vi "ManualScan-V17.vi"(8 "Button-OK":bool, 10 "menu reference":refnum<k9>, 11 "SN Length":string) -> (1 "MainProcess":T1, 3 "Barcode out:":string)   [LabVIEW 2013]
uses:
  Control/SystemProcess.ctl
  <vilib>/Utility/error.llb/whitespace.ctl
  <vilib>/event_ctls.llb/eventvkey.ctl
  Control/Buffer.vi
panel:
  in  "Button-Cancel":bool
  in  "Barcode(S/N):":string
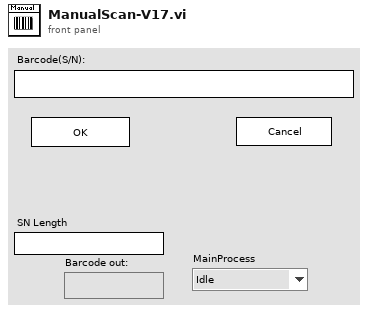
[diagram p1: front panel]
types:
  T1 = typedef "SystemProcess.ctl" = enum16{"Idle", "SystemInit", "SpecialEvent", "Barcode(SN)", "TestInitialize", "Test", "Stop", "SaveTestData", "Exit"}
  T2 = typedef "eventvkey.ctl" = enum16{"ASCII", "Enter", "Return", "Shift", "Ctrl", "Alt", "Cmd", "Opt", "Caps", "NumLock", "Clear", "Break", "Up", "Down", "Left", "Right", "Insert", "Delete", "Home", "End", "PageUp", "PageDown", "Escape", "Help", "Pause", "ScrollLock", "F1", "F2", "F3", "F4", "F5", "F6", "F7", "F8", "F9", "F10", "F11", "F12", "F13", "F14", "F15", "F16", "F17", "F18", "F19", "F20", "F21", "F22", "F23", "F24", "Play", "VolumeUp", "VolumeDown", "Mute", "Two Byte Char"}
  T3 = typedef "whitespace.ctl" = u16
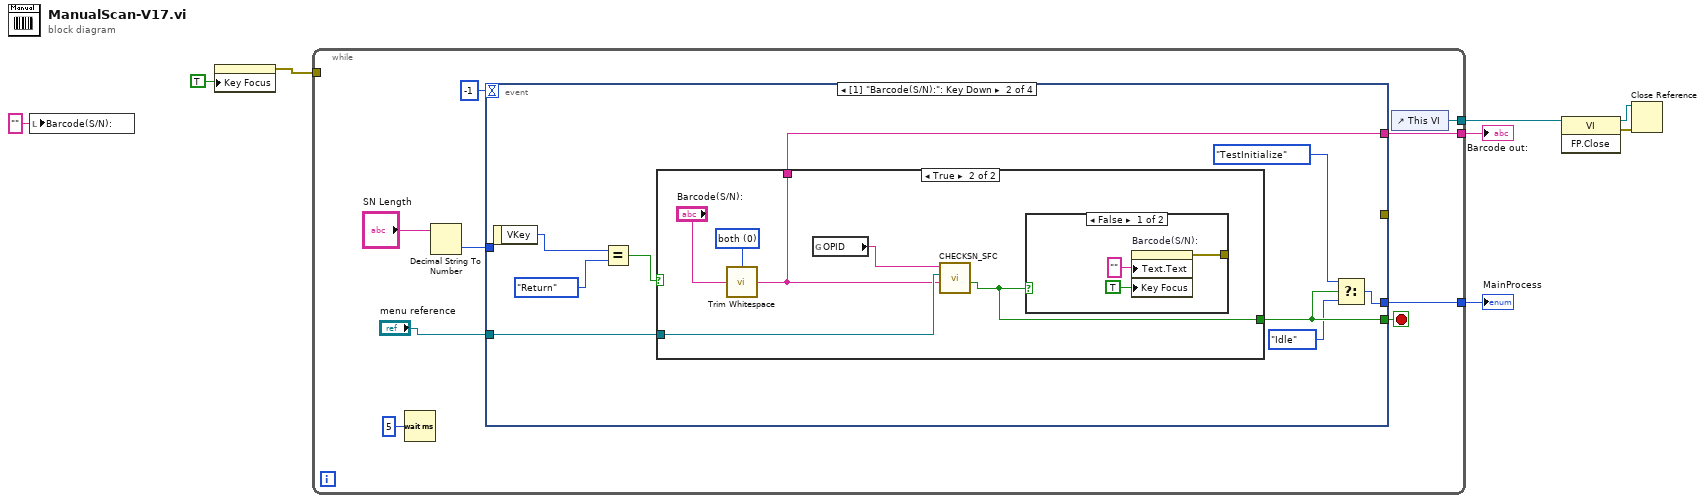
[diagram p0: block diagram]
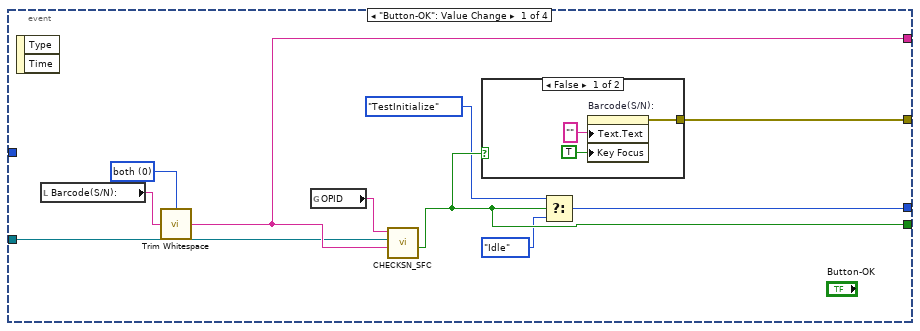
[diagram p2: hidden frame]
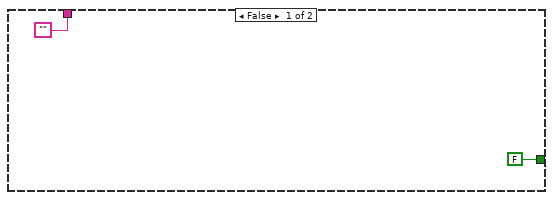
[diagram p4: hidden frame]
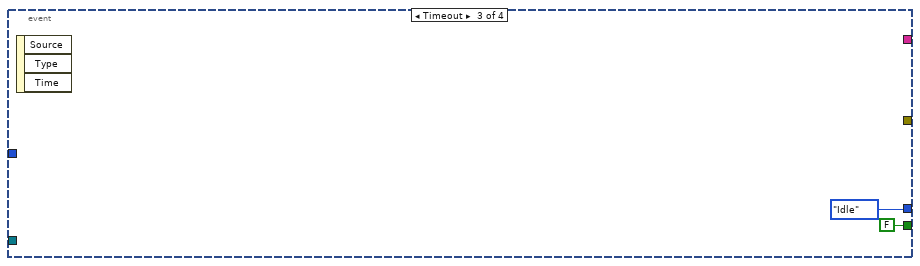
[diagram p6: hidden frame]
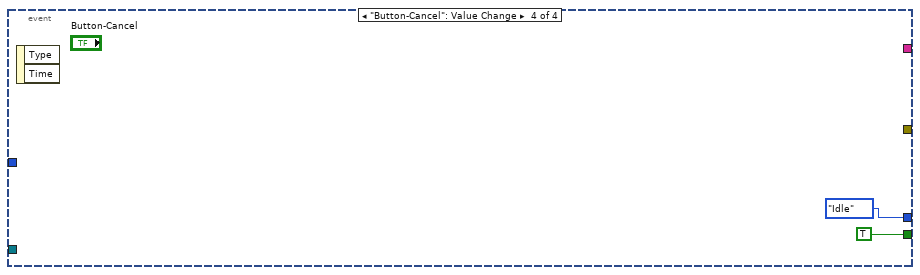
[diagram p7: hidden frame]
diagram:
  n1 = local write "Barcode(S/N):"("" ("Barcode(S/N):")) -> ()
  n2 = property on="Barcode(S/N):" class="Str"("Key Focus"=TRUE) -> (error out=w3:errorcluster)  [unwired: 2 in, 1 out]
  n3 = while {
    tunnel: [w17] -> w5
    tunnel: [w16] -> w4
    tunnel: w3 -> [_]
    tunnel: [w14] -> w2
    stop <- w15 stop-if-true
    n4 = Wait (ms)(milliseconds to wait=u32 5) -> ()  [unwired: 1 out]
    n5 = Decimal String To Number(string="SN Length") -> (number=w11:i32)  [unwired: 2 in, 1 out]
    n6 = event shown="[1] \"Barcode(S/N):\": Key Down" {
      selector: _ -> [_ _ _ _]
      dyn-events: _ -> [_ _ _ _]
      timeout: -1 -> [_ _ _ _]
      tunnel: [w26 w34 FALSE ("OK in") TRUE ("OK in")] -> w15
      tunnel: [w24 w36 _ _] -> w16
      tunnel: [w27 w32 SystemProcess."Idle" ("MainProcess") SystemProcess."Idle" ("MainProcess")] -> w14
      tunnel: [w25 _ _ _] -> _
      tunnel: w11 -> [_ _ _ _]
      tunnel: "menu reference" -> [w18 w35 _ _]
      event "Button-OK": Value Change {
        w19 = T3 0 items=["both", "start of string", "end of string"] ("location (both)")
        n7 = event-data() -> ()  [unwired: 1 in, 2 out]
        n8 = local read "Barcode(S/N):"() -> (w20:string)
        n9 = call <vilib>:"Trim Whitespace.vi"("string"=w20, "location (both)"=w19) -> ("trimmed string"=w24:string)
        n10 = global read "Buffer.vi" "OPID"() -> (w21:string)
        n11 = call "CHECKSN_SFC.vi"("SN"=w24, "menu reference"=w18, "OPID"=w21) -> ("SNCheck"=w26:bool)  [unwired: 7 in, 1 out]
        n12 = case shown="False" w26 {
          tunnel: [w28 _] -> w25
          frame False {
            n13 = property on="Barcode(S/N):" class="Str"("Text.Text"="", "Key Focus"=TRUE) -> (error out=w28:errorcluster)  [unwired: 2 in, 1 out]
          }
          frame True {
          }
        }
        n14 = Select(t=SystemProcess."TestInitialize" ("MainProcess"), s=w26, f=SystemProcess."Idle") -> (s? t:f=w27:T1)
      }
      event "Barcode(S/N):": Key Down {
        n15 = event-data() -> ("VKey"=w39:T2)  [unwired: 1 in]
        n16 = Equal?(x=w39, y=eventvkey."Return" ("VKey")) -> (x = y?=w37:bool)
        n17 = case shown="True" w37 {
          tunnel: ["" w43] -> w36
          tunnel: [FALSE w45] -> w34
          tunnel: w35 -> [_ w44]
          frame False {
          }
          frame True {
            w42 = T3 0 items=["both", "start of string", "end of string"] ("location (both)")
            n18 = call <vilib>:"Trim Whitespace.vi"("string"="Barcode(S/N):", "location (both)"=w42) -> ("trimmed string"=w43:string)
            n19 = global read "Buffer.vi" "OPID"() -> (w47:string)
            n20 = call "CHECKSN_SFC.vi"("SN"=w43, "menu reference"=w44, "OPID"=w47) -> ("SNCheck"=w45:bool)  [unwired: 7 in, 1 out]
            n21 = case shown="False" w45 {
              tunnel: [w48 _] -> _
              frame False {
                n22 = property on="Barcode(S/N):" class="Str"("Text.Text"="", "Key Focus"=TRUE) -> (error out=w48:errorcluster)  [unwired: 2 in, 1 out]
              }
              frame True {
              }
            }
          }
        }
        n23 = Select(t=SystemProcess."TestInitialize" ("MainProcess"), s=w34, f=SystemProcess."Idle" ("MainProcess")) -> (s? t:f=w32:T1)
      }
      event Timeout {
        n24 = event-data() -> ()  [unwired: 1 in, 3 out]
      }
      event "Button-Cancel": Value Change {
        n25 = event-data() -> ()  [unwired: 1 in, 2 out]
      }
    }
    n26 = control-ref of="This VI"() -> (w17:refnum<vi>)
  }
  "Barcode out:" <- w4
  "MainProcess" <- w2
  n27 = invoke class="VI" method="FP.Close"(reference=w5) -> (reference out=w7:refnum<vi>, error out=w6:errorcluster)  [unwired: 2 in, 1 out]
  n28 = Close Reference(reference=w7, error in (no error)=w6) -> ()  [unwired: 1 out]
